vi "DSF.Engine.Framework.Get Cache.vi"(11 "Framework in":refnum<class "DSF.Engine.Framework.lvclass">) -> (2 "Cache":refnum<class "DSF.Engine.Memory.Cache.lvclass">, 3 "Framework out":refnum<class "DSF.Engine.Framework.lvclass">)   [LabVIEW 2017, in "DSF.Engine.lvlib" / "DSF.Engine.Framework.lvclass"]
uses:
  DSF.Engine.Framework.lvclass
  Cache/DSF.Engine.Memory.Cache.lvclass
  DSF.Engine.Framework.lvclass/DSF.Engine.Framework.ctl
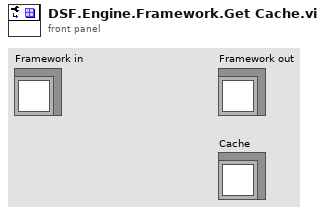
[diagram p1: front panel]
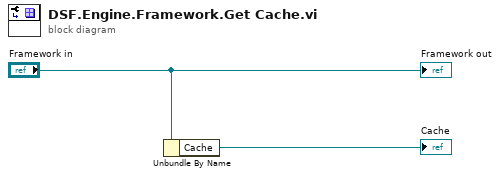
[diagram p0: block diagram]
diagram:
  n1 = Unbundle By Name("Framework in") -> ("Cache"=→"Cache":refnum<class "DSF.Engine.Memory.Cache.lvclass">)
  "Framework out" <- "Framework in"
